vi "Exemple2DClassification.vi"() -> ()   [LabVIEW 2020]
uses:
  _Controls/PointPropertyMultipleLabel.ctl
  _Controls/Style.ctl
  Controls/2DParameters.ctl
  _Controls/Datas.ctl
panel:
  in  "Predict":dbl[][](array[numeric])=[[0.0], [0.0], [0.0], [0.0], [0.0], [0.0], [0.0], [0.0], [0.0], [0.0], [0.0], [0.0], [0.0], [0.0], [0.0], [0.0], [0.0], [0.0], [0.0], [0.0], [0.0], [0.0], [0.0], [0.0], [0.0], [0.0], [1.0], [1.0], [1.0], [1.0], [1.0], [1.0], [1.0], [1.0], [1.0], [1.0], [1.0], [1.0], [2.0], [1.0], [1.0], [1.0], [1.0], [1.0], [1.0], [1.0], [1.0], [1.0], [1.0], [1.0], [1.0], [2.0], [2.0], [2.0], [2.0], [2.0], [2.0], [2.0], [2.0], [2.0], [2.0], [2.0], [2.0], [2.0], [2.0], [2.0], [2.0], [2.0], [2.0], [2.0], [2.0], [2.0], [2.0], [2.0], [2.0]]
  in  "Split":T1={"X Train"=[[5.1, 3.5, 1.4, 0.2], [4.9, 3.0, 1.4, 0.2], [4.7, 3.2, 1.3, 0.2], [5.0, 3.6, 1.4, 0.2], [4.6, 3.4, 1.4, 0.3], [5.0, 3.4, 1.5, 0.2], [5.7, 4.4, 1.5, 0.4], [5.1, 3.5, 1.4, 0.3], [5.1, 3.7, 1.5, 0.4], [5.0, 3.0, 1.6, 0.2], [5.0, 3.4, 1.6, 0.4], [4.7, 3.2, 1.6, 0.2], [5.4, 3.4, 1.5, 0.4], [5.2, 4.1, 1.5, 0.1], [4.9, 3.1, 1.5, 0.2], [5.0, 3.2, 1.2, 0.2], [4.9, 3.6, 1.4, 0.1], [4.4, 3.0, 1.3, 0.2], [4.5, 2.3, 1.3, 0.3], [5.0, 3.5, 1.6, 0.6], [5.1, 3.8, 1.9, 0.4], [4.8, 3.0, 1.4, 0.3], [4.6, 3.2, 1.4, 0.2], [5.3, 3.7, 1.5, 0.2], [7.0, 3.2, 4.7, 1.4], [5.5, 2.3, 4.0, 1.3], [6.5, 2.8, 4.6, 1.5], [5.2, 2.7, 3.9, 1.4], [6.0, 2.2, 4.0, 1.0], [5.6, 2.9, 3.6, 1.3], [5.6, 3.0, 4.5, 1.5], [5.8, 2.7, 4.1, 1.0], [6.1, 2.8, 4.0, 1.3], [6.3, 2.5, 4.9, 1.5], [6.4, 2.9, 4.3, 1.3], [6.6, 3.0, 4.4, 1.4], [6.0, 2.9, 4.5, 1.5], [5.5, 2.4, 3.7, 1.0], [6.0, 2.7, 5.1, 1.6], [5.4, 3.0, 4.5, 1.5], [6.0, 3.4, 4.5, 1.6], [6.7, 3.1, 4.7, 1.5], [5.5, 2.6, 4.4, 1.2], [5.8, 2.6, 4.0, 1.2], [5.0, 2.3, 3.3, 1.0], [5.7, 3.0, 4.2, 1.2], [5.7, 2.9, 4.2, 1.3], [5.1, 2.5, 3.0, 1.1], [5.7, 2.8, 4.1, 1.3], [6.3, 3.3, 6.0, 2.5], [5.8, 2.7, 5.1, 1.9], [6.3, 2.9, 5.6, 1.8], [7.6, 3.0, 6.6, 2.1], [7.2, 3.6, 6.1, 2.5], [6.5, 3.2, 5.1, 2.0], [6.4, 2.7, 5.3, 1.9], [6.8, 3.0, 5.5, 2.1], [6.4, 3.2, 5.3, 2.3], [6.5, 3.0, 5.5, 1.8], [6.0, 2.2, 5.0, 1.5], [6.3, 2.7, 4.9, 1.8], [6.7, 3.3, 5.7, 2.1], [6.1, 3.0, 4.9, 1.8], [7.4, 2.8, 6.1, 1.9], [6.4, 2.8, 5.6, 2.2], [6.3, 2.8, 5.1, 1.5], [7.7, 3.0, 6.1, 2.3], [6.4, 3.1, 5.5, 1.8], [6.0, 3.0, 4.8, 1.8], [6.7, 3.1, 5.6, 2.4], [6.9, 3.1, 5.1, 2.3], [6.8, 3.2, 5.9, 2.3], [6.7, 3.3, 5.7, 2.5], [6.3, 2.5, 5.0, 1.9], [6.2, 3.4, 5.4, 2.3]], "X Test"=[[4.6, 3.1, 1.5, 0.2], [5.4, 3.9, 1.7, 0.4], [4.4, 2.9, 1.4, 0.2], [4.9, 3.1, 1.5, 0.1], [5.4, 3.7, 1.5, 0.2], [4.8, 3.4, 1.6, 0.2], [4.8, 3.0, 1.4, 0.1], [4.3, 3.0, 1.1, 0.1], [5.8, 4.0, 1.2, 0.2], [5.4, 3.9, 1.3, 0.4], [5.7, 3.8, 1.7, 0.3], [5.1, 3.8, 1.5, 0.3], [5.4, 3.4, 1.7, 0.2], [4.6, 3.6, 1.0, 0.2], [5.1, 3.3, 1.7, 0.5], [4.8, 3.4, 1.9, 0.2], [5.2, 3.5, 1.5, 0.2], [5.2, 3.4, 1.4, 0.2], [4.8, 3.1, 1.6, 0.2], [5.5, 4.2, 1.4, 0.2], [5.5, 3.5, 1.3, 0.2], [5.1, 3.4, 1.5, 0.2], [5.0, 3.5, 1.3, 0.3], [4.4, 3.2, 1.3, 0.2], [5.1, 3.8, 1.6, 0.2], [5.0, 3.3, 1.4, 0.2], [6.4, 3.2, 4.5, 1.5], [6.9, 3.1, 4.9, 1.5], [5.7, 2.8, 4.5, 1.3], [6.3, 3.3, 4.7, 1.6], [4.9, 2.4, 3.3, 1.0], [6.6, 2.9, 4.6, 1.3], [5.0, 2.0, 3.5, 1.0], [5.9, 3.0, 4.2, 1.5], [6.1, 2.9, 4.7, 1.4], [6.7, 3.1, 4.4, 1.4], [6.2, 2.2, 4.5, 1.5], [5.6, 2.5, 3.9, 1.1], [5.9, 3.2, 4.8, 1.8], [6.1, 2.8, 4.7, 1.2], [6.8, 2.8, 4.8, 1.4], [6.7, 3.0, 5.0, 1.7], [5.7, 2.6, 3.5, 1.0], [5.5, 2.4, 3.8, 1.1], [5.8, 2.7, 3.9, 1.2], [6.3, 2.3, 4.4, 1.3], [5.6, 3.0, 4.1, 1.3], [5.5, 2.5, 4.0, 1.3], [6.1, 3.0, 4.6, 1.4], [5.6, 2.7, 4.2, 1.3], [6.2, 2.9, 4.3, 1.3], [7.1, 3.0, 5.9, 2.1], [6.5, 3.0, 5.8, 2.2], [4.9, 2.5, 4.5, 1.7], [7.3, 2.9, 6.3, 1.8], [6.7, 2.5, 5.8, 1.8], [5.7, 2.5, 5.0, 2.0], [5.8, 2.8, 5.1, 2.4], [7.7, 3.8, 6.7, 2.2], [7.7, 2.6, 6.9, 2.3], [6.9, 3.2, 5.7, 2.3], [5.6, 2.8, 4.9, 2.0], [7.7, 2.8, 6.7, 2.0], [7.2, 3.2, 6.0, 1.8], [6.2, 2.8, 4.8, 1.8], [6.4, 2.8, 5.6, 2.1], [7.2, 3.0, 5.8, 1.6], [7.9, 3.8, 6.4, 2.0], [6.1, 2.6, 5.6, 1.4], [6.3, 3.4, 5.6, 2.4], [6.9, 3.1, 5.4, 2.1], [5.8, 2.7, 5.1, 1.9], [6.7, 3.0, 5.2, 2.3], [6.5, 3.0, 5.2, 2.0], [5.9, 3.0, 5.1, 1.8]], "Y Train"=[[0.0], [0.0], [0.0], [0.0], [0.0], [0.0], [0.0], [0.0], [0.0], [0.0], [0.0], [0.0], [0.0], [0.0], [0.0], [0.0], [0.0], [0.0], [0.0], [0.0], [0.0], [0.0], [0.0], [0.0], [1.0], [1.0], [1.0], [1.0], [1.0], [1.0], [1.0], [1.0], [1.0], [1.0], [1.0], [1.0], [1.0], [1.0], [1.0], [1.0], [1.0], [1.0], [1.0], [1.0], [1.0], [1.0], [1.0], [1.0], [1.0], [2.0], [2.0], [2.0], [2.0], [2.0], [2.0], [2.0], [2.0], [2.0], [2.0], [2.0], [2.0], [2.0], [2.0], [2.0], [2.0], [2.0], [2.0], [2.0], [2.0], [2.0], [2.0], [2.0], [2.0], [2.0], [2.0]], "Y Test"=[[0.0], [0.0], [0.0], [0.0], [0.0], [0.0], [0.0], [0.0], [0.0], [0.0], [0.0], [0.0], [0.0], [0.0], [0.0], [0.0], [0.0], [0.0], [0.0], [0.0], [0.0], [0.0], [0.0], [0.0], [0.0], [0.0], [1.0], [1.0], [1.0], [1.0], [1.0], [1.0], [1.0], [1.0], [1.0], [1.0], [1.0], [1.0], [1.0], [1.0], [1.0], [1.0], [1.0], [1.0], [1.0], [1.0], [1.0], [1.0], [1.0], [1.0], [1.0], [2.0], [2.0], [2.0], [2.0], [2.0], [2.0], [2.0], [2.0], [2.0], [2.0], [2.0], [2.0], [2.0], [2.0], [2.0], [2.0], [2.0], [2.0], [2.0], [2.0], [2.0], [2.0], [2.0], [2.0]]}
  in  "Display":T2={"Choice"=enum."All", "Indexe"={"X"=0, "Y"=1}}
  in  "Point Property":T3={"Train Style"=enum."Full circle", "Test OK Style"=enum."Full square", "Label Color"=[8978528, 4367871, 1985280], "Test NO OK"={"Style"=enum."Cross", "Color"=16716800}}
  out "error out":errorcluster
  in  "error in":errorcluster
  out "Plot":cluster{"X":dbl[], "Y":dbl[]}[](graph)
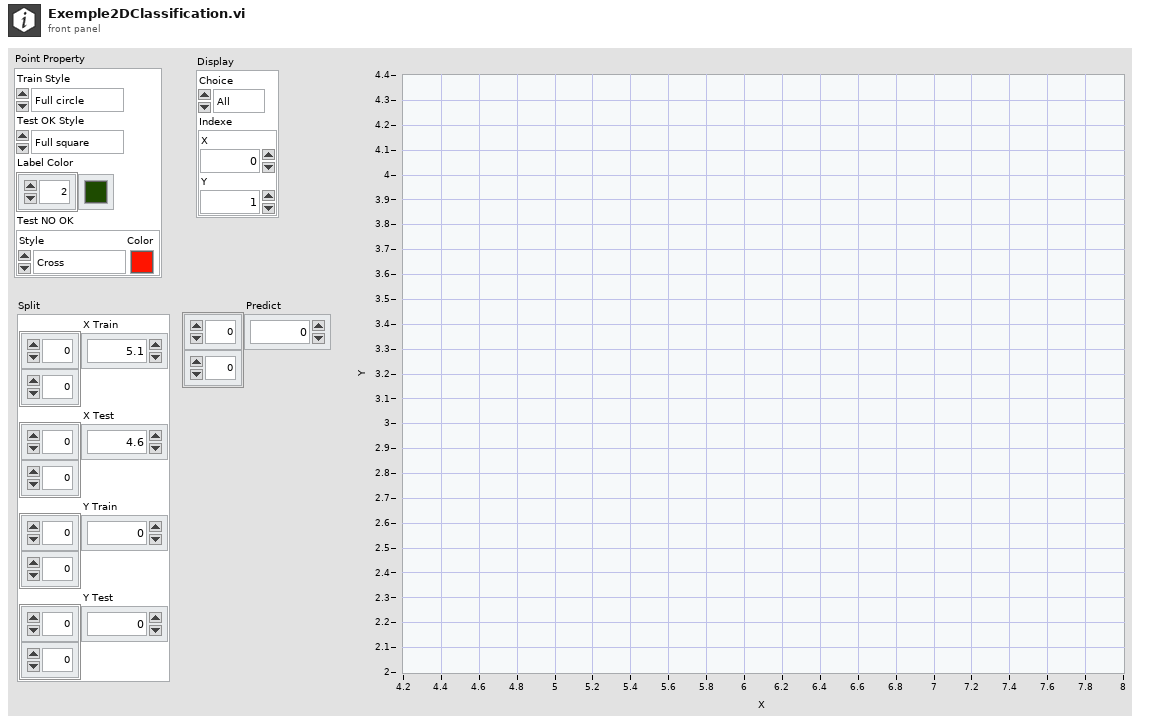
[diagram p1: front panel]
types:
  T1 = cluster{"X Train":dbl[][], "X Test":dbl[][], "Y Train":dbl[][], "Y Test":dbl[][]}
  T2 = cluster{"Choice":enum16{"All", "Train", "Test"}, "Indexe":cluster{"X":i32, "Y":i32}}
  T3 = typedef "PointPropertyMultipleLabel.ctl" = cluster{"Train Style":T4, "Test OK Style":T4, "Label Color":u32[], "Test NO OK":cluster{"Style":T4, "Color":u32}}
  T4 = typedef "Style.ctl" = enum16{"Empty circle", "Full circle", "Empty square", "Full square", "Cross"}
  T5 = typedef "2DParameters.ctl" = cluster{"Plot":refnum<vi>, "Data":T6, "Display":cluster{"Choice":enum16{"All", "Train", "Test"}, "Indexe":cluster{"X":i32, "Y":i32}}, "Property":T3}
  T6 = typedef "Datas.ctl" = cluster{"Split":cluster{"X Train":dbl[][], "X Test":dbl[][], "Y Train":dbl[][], "Y Test":dbl[][]}, "Predict":dbl[][]}
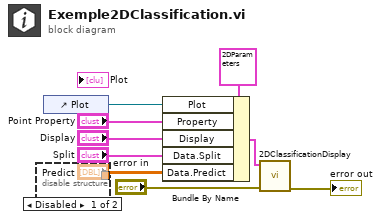
[diagram p0: block diagram]
diagram:
  n1 = disable-structure shown="Disabled" {
    disable-tunnel: ["Predict" _] -> w9
    frame Disabled {
    }
    frame Enabled {
    }
  }
  n2 = control-ref of="Plot"() -> (w3:refnum<vi>)
  n3 = Bundle By Name(cluster=T5 {"Plot"=refnum, "Data"={"Split"={"X Train"=[], "X Test"=[], "Y Train"=[], "Y Test"=[]}, "Predict"=[]}, "Display"={"Choice"=enum."All", "Indexe"={"X"=0, "Y"=1}}, "Property"={"Train Style"=enum."Full circle", "Test OK Style"=enum."Full square", "Label Color"=[8978528, 4367871, 1985280], "Test NO OK"={"Style"=enum."Cross", "Color"=16716800}}} ("Parameters"), "Plot"=w3, "Property"="Point Property", "Display"="Display", "Data.Split"="Split", "Data.Predict"=w9) -> (w2:T5)
  n4 = call "2DClassificationDisplay.vi"("error in"="error in", "Parameters"=w2) -> ("error out"=→"error out":errorcluster)  [unwired: 9 in]
